vi "cos wave.vi"(6 "phi":dbl, 9 "f":dbl, 10 "dt":dbl, 11 "N":i32) -> (1 "cos wt":waveform(dbl))   [LabVIEW 2013]
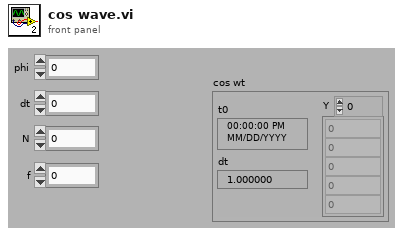
[diagram p1: front panel]
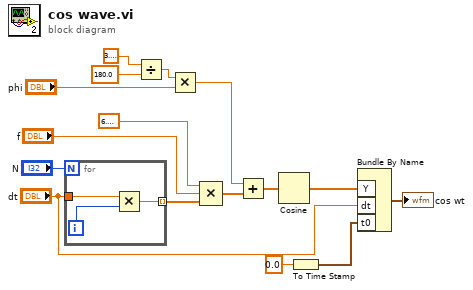
[diagram p0: block diagram]
diagram:
  n1 = for {
    N: "N" -> [_]
    tunnel: "dt" -> [w18]
    tunnel: [w17] -> w12 mode=indexing
    i -> [w19]
    n2 = Multiply(x=w18, y=w19) -> (x*y=w17:dbl)
  }
  n3 = Divide(x=3.141592653589793, y=180.0) -> (x/y=w1:dbl)
  n4 = Multiply(x=w1, y="phi") -> (x*y=w2:dbl)
  n5 = Compound Arithmetic op=MULTIPLY(6.283185307179586, "f", w12) -> (w6:dbl[])
  n6 = Add(x=w2, y=w6) -> (x+y=w5:dbl[])
  n7 = Cosine(x=w5) -> (cos(x)=w14:dbl[])
  n8 = To Time Stamp(1:0.0) -> (0:w9:timestamp)
  n9 = Bundle By Name("Y"=w14, "dt"="dt", "t0"=w9) -> (→"cos wt":waveform(dbl))  [unwired: 1 out]
